vi "ConnectToDB.vi"(8 "Error In":errorcluster, 11 "UDL_Path":path) -> (0 "Error Out":errorcluster, 2 "dup UDL_Path":path, 3 "Refnum out":T1)   [LabVIEW 2020]
uses:
  <vilib>/addons/database/Connection.llb/Conn ObjectReference.ctl
  <vilib>/addons/database/Connection.llb/DB Tools Open Connec (Path).vi
  <vilib>/addons/database/NI_Database_API.lvlib
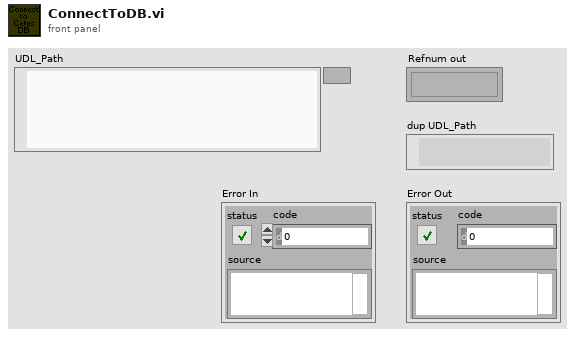
[diagram p1: front panel]
types:
  T1 = typedef "NI_Database_API.lvlib/Conn ObjectReference.ctl" = refnum<k1>
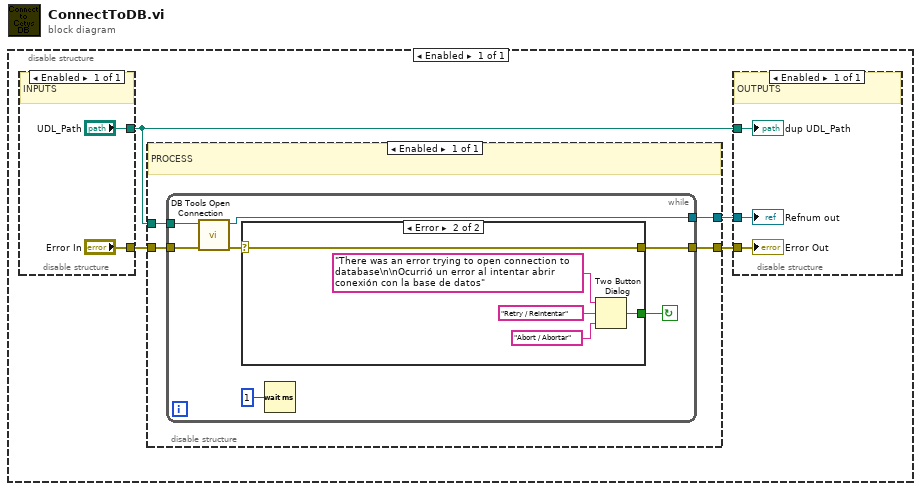
[diagram p0: block diagram]
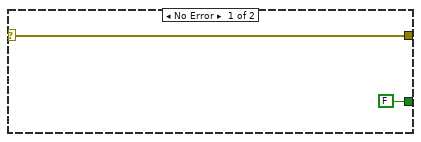
[diagram p2: hidden frame]
diagram:
  n1 = disable-structure shown="Enabled" {
    frame Enabled {
      n2 = disable-structure shown="Enabled" {
        disable-tunnel: ["Error In"] -> w4
        disable-tunnel: ["UDL_Path"] -> w1
        frame Enabled {
          # "INPUTS"
        }
      }
      n3 = disable-structure shown="Enabled" {
        disable-tunnel: w4 -> [w8]
        disable-tunnel: [w7] -> w3
        disable-tunnel: [w6] -> w2
        disable-tunnel: w1 -> [w5]
        frame Enabled {
          # "PROCESS"
          n4 = while {
            tunnel: [w15] -> w6
            tunnel: w5 -> [w14]
            tunnel: w8 -> [w13]
            tunnel: [w9] -> w7
            stop <- w12 continue-if-true
            n5 = call-poly <vilib>:"DB Tools Open Connection.vi"("error in (no error)"=w13, "connection information"=w14) -> ("error out"=w10:errorcluster, "connection reference"=w15:T1)  [unwired: 6 in]
            n6 = case shown="Error" w10 {
              selector: w10 -> [w16 w19]
              tunnel: [FALSE w18] -> w12
              tunnel: [w16 w19] -> w9
              frame No Error {
              }
              frame Error {
                n7 = Two Button Dialog(message="There was an error trying to open connection to database\n\nOcurrió un error al intentar abrir conexión con la base de datos", 1:"Abort / Abortar" ("F button name (\"Cancel\")"), 2:"Retry / Reintentar" ("T button name (\"OK\")")) -> (T button?=w18:bool)
              }
            }
            n8 = Wait (ms)(milliseconds to wait=u32 1) -> ()  [unwired: 1 out]
          }
        }
      }
      n9 = disable-structure shown="Enabled" {
        disable-tunnel: w3 -> [w27]
        disable-tunnel: w2 -> [w26]
        disable-tunnel: w1 -> [w25]
        frame Enabled {
          # "OUTPUTS"
          "Error Out" <- w27
          "Refnum out" <- w26
          "dup UDL_Path" <- w25
        }
      }
    }
  }
